vi "SetSnakeRef.vi"(8 "Error In":errorcluster, 10 "SnakeRef":refnum<class "Snake.lvclass">, 11 "object in":refnum<class "Board Game.lvclass">) -> (0 "Error Out":errorcluster, 3 "object out":refnum<class "Board Game.lvclass">)   [LabVIEW 2021, in "Board Game.lvclass"]
uses:
  Board Game.lvclass
  Snake_class/Snake.lvclass
  C:/Users/poche/Programs/LabVIEW/imposible snake/GameEl_class/GameEl.lvclass
  Board Game.lvclass/Board Game.ctl
  GameEl_class/GameEl.lvclass/GameEl.ctl
  GameEl_class/Read Colour.vi
  GameEl_class/Read position.vi
  GameEl_class/GameEl.lvclass
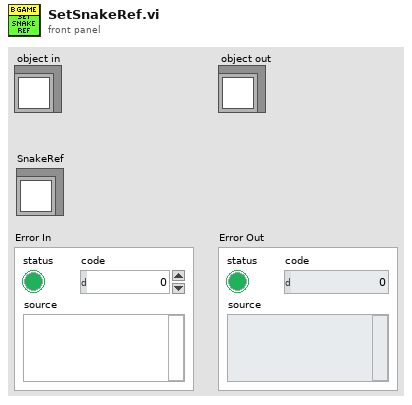
[diagram p1: front panel]
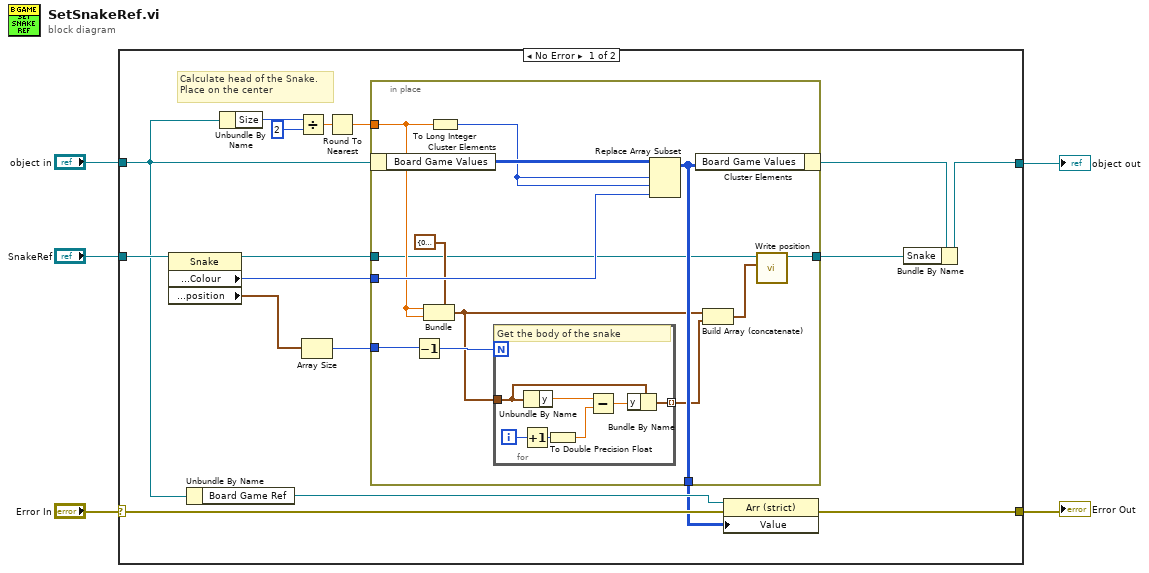
[diagram p0: block diagram]
diagram:
  n1 = case shown="No Error" "Error In" {
    selector: "Error In" -> [w21 w44]
    tunnel: [w15 w44] -> w4
    tunnel: [w10 w43] -> w2
    tunnel: "object in" -> [w12 w43]
    tunnel: "SnakeRef" -> [w22 _]
    frame No Error {
      # "Calculate head of the Snake. \nPlace on the center"
      n2 = property class="Snake"(reference=w22) -> (reference out=w9:refnum<class "Snake.lvclass">, "SubVIs:DataAccess:Colour"=w16:u32, "SubVIs:DataAccess:position"=w7:cluster{"x":dbl, "y":dbl}[])  [unwired: 1 in, 1 out]
      n3 = Unbundle By Name(w12) -> ("Board Game Ref"=w14:refnum<vi>)
      n4 = Unbundle By Name(w12) -> ("Size"=w20:u16)
      n5 = Divide(x=w20, y=u16 2) -> (x/y=w18:dbl)
      n6 = Array Size(array=w7) -> (size(s)=w6:i32)
      n7 = Round To Nearest(number=w18) -> (nearest integer value=w17:dbl)
      n8 = in-place {
        in-place-border: w17 -> [w31]
        in-place-border: w16 -> [w33]
        in-place-border: [w32] -> w13
        in-place-border: w9 -> [w25]
        in-place-border: [w23] -> w8
        in-place-border: w6 -> [w30]
        n9 = in-place-cluster #1(w12) -> ("Board Game Values"=w35:u32[][])
        n10 = Decrement(x=w30) -> (x-1=w29:i32)
        n11 = Bundle(cluster=cluster{"x":dbl, "y":dbl} {"x"=0.0, "y"=0.0}, "x"=w31, "y"=w31) -> (w28:cluster{"x":dbl, "y":dbl})
        n12 = To Long Integer(number=w31) -> (32bit integer=w34:i32)
        n13 = for {
          N: w29 -> [_]
          tunnel: w28 -> [w38]
          tunnel: [w36] -> w26 mode=indexing
          i -> [w42]
          # "Get the body of the snake"
          n14 = Increment(x=w42) -> (x+1=w40:i32)
          n15 = Unbundle By Name(w38) -> ("y"=w41:dbl)
          n16 = To Double Precision Float(number=w40) -> (double precision float=w39:dbl)
          n17 = Subtract(x=w41, y=w39) -> (x-y=w37:dbl)
          n18 = Bundle By Name(cluster=w38, "y"=w37) -> (w36:cluster{"x":dbl, "y":dbl})
        }
        n19 = Replace Array Subset(array=w35, new element=w33, index (row)=w34, index (col)=w34) -> (w32:u32[][])
        n20 = in-place-cluster #1("Board Game Values"=w32) -> (w11:refnum<class "Board Game.lvclass">)
        n21 = Build Array (concatenate)(w28, w26) -> (w24:cluster{"x":dbl, "y":dbl}[])
        n22 = call "Write position.vi"("position"=w24, "GameEl in"=w25) -> ("GameEl out"=w23:refnum<class "Snake.lvclass">)  [unwired: 8 in, 1 out]
      }
      n23 = property class="Arr (strict)"(reference=w14, error in=w21, "Value"=w13) -> (error out=w15:errorcluster)  [unwired: 1 out]
      n24 = Bundle By Name(cluster=w11, "Snake"=w8) -> (w10:refnum<class "Board Game.lvclass">)
    }
    frame Error {
    }
  }
  "Error Out" <- w4
  "object out" <- w2
